vi "Write Ramp Parameters.vi"(8 "error in (no error)":errorcluster, 9 "low":dbl, 10 "high":dbl, 11 "Ramp Setpoint in":refnum<class "Ramp Setpoint.lvclass">) -> (0 "error out":errorcluster, 3 "Ramp Setpoint out":refnum<class "Ramp Setpoint.lvclass">)   [LabVIEW 2020, in "Ramp Setpoint.lvclass"]
uses:
  Ramp Setpoint.lvclass
  Ramp Setpoint.lvclass/Ramp Setpoint.ctl
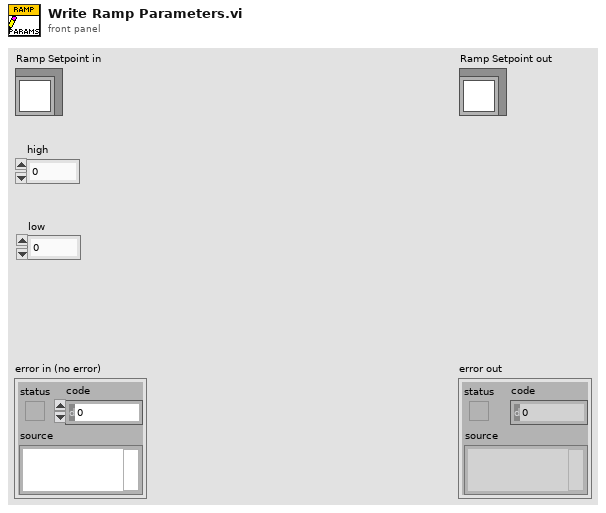
[diagram p1: front panel]
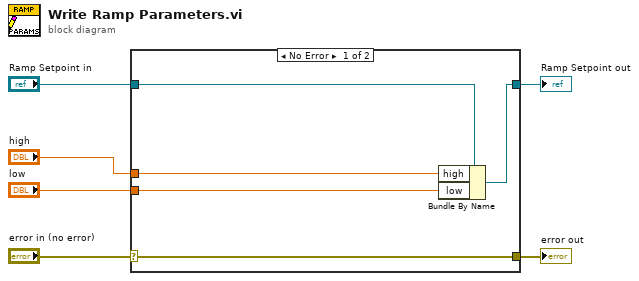
[diagram p0: block diagram]
diagram:
  n1 = case shown="No Error" "error in (no error)" {
    selector: "error in (no error)" -> [w11 w12]
    tunnel: [w11 w12] -> w5
    tunnel: [w9 w13] -> w3
    tunnel: "Ramp Setpoint in" -> [w10 w13]
    tunnel: "high" -> [w8 _]
    tunnel: "low" -> [w7 _]
    frame No Error {
      n2 = Bundle By Name(cluster=w10, "high"=w8, "low"=w7) -> (w9:refnum<class "Ramp Setpoint.lvclass">)
    }
    frame Error {
    }
  }
  "error out" <- w5
  "Ramp Setpoint out" <- w3
